vi "OP500Z8_SCANequipements.vi"(8 "Errin":errorcluster caption="errin", 10 "Chaîne":string="Log et conf\\Config.ini", 11 "pathin":path=path "D:/CODE/02 SLIM ZEN") -> (0 "errout":errorcluster={"status"=TRUE, "code"=0, "source"="PCAN_CHANNEL ILLEGAL"}, 1 "KO?":bool=TRUE, 3 "VISA OUT":T1)   [LabVIEW 2020]
doc: "Ce vi il détecte la presence des équipements"
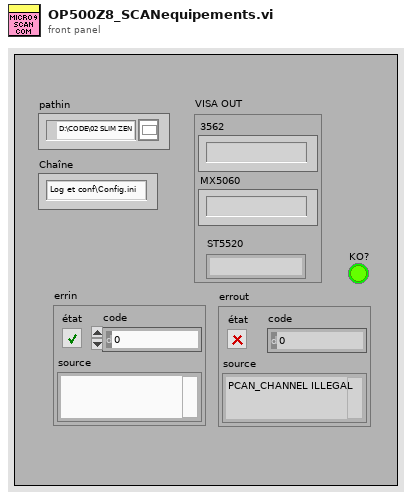
[diagram p1: front panel]
types:
  T1 = cluster{"3562":string, "MX5060":string, "ST5520":string}
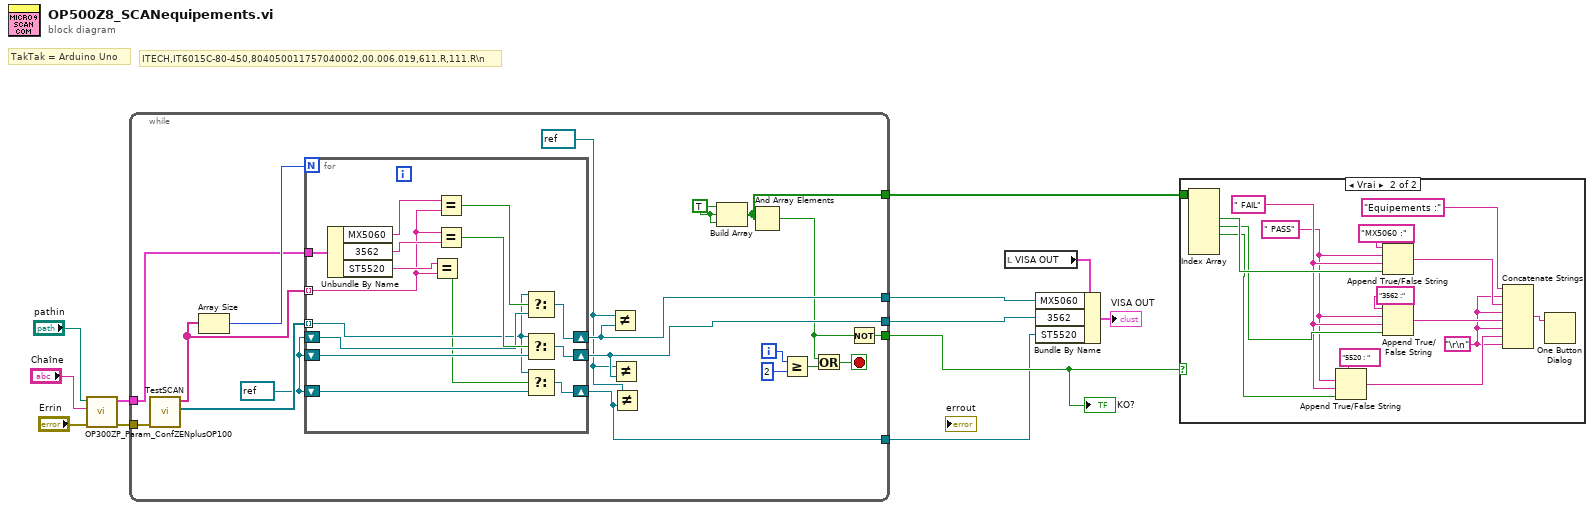
[diagram p0: block diagram]
diagram:
  # "TakTak = Arduino Uno"
  # "ITECH,IT6015C-80-450,804050011757040002,00.006.019,611.R,111.R\\n"
  n1 = call "OP300ZP_Param_ConfZENplusOP100.vi"("errin"="Errin", "Chaîne"="Chaîne", "pathin"="pathin") -> ("errout"=w7:errorcluster, "VISA OUT"=w6:T1)  [unwired: 7 in]
  n2 = while {
    tunnel: [w20] -> w12
    tunnel: [w19] -> w11
    tunnel: w7 -> [w29]
    tunnel: [w24] -> w10
    tunnel: w6 -> [w21]
    tunnel: [w17] -> w9
    tunnel: [w14] -> w1
    i -> [w23]
    stop <- w26 stop-if-true
    w13 = TRUE ("élément")
    w15 = refnum<visa-resource-name> refnum ("x")
    w16 = refnum<visa-resource-name> refnum ("VISA resource name out")
    n3 = call "TestSCAN.vi"("errin"=w29) -> ("Tableau 2"=w27:refnum<visa-resource-name>[], "Tableau"=w28:string[])  [unwired: 8 in, 1 out]
    n4 = Array Size(array=w28) -> (size(s)=w30:i32)
    n5 = for {
      N: w30 -> [_]
      shift-right: [w43] -> w20
      shift-left: w16 -> [w41]
      shift-right: [w42] -> w19
      shift-left: w16 -> [w40]
      tunnel: w28 -> [w32] mode=indexing
      tunnel: w21 -> [w39]
      shift-right: [w35] -> w14
      shift-left: w16 -> [w36]
      tunnel: w27 -> [w34] mode=indexing
      n6 = Unbundle By Name(w39) -> ("MX5060"=w38:string, "3562"=w37:string, "ST5520"=w33:string)
      n7 = Equal?(x=w33, y=w32) -> (x = y?=w31:bool)
      n8 = Equal?(x=w38, y=w32) -> (x = y?=w44:bool)
      n9 = Equal?(x=w32, y=w37) -> (x = y?=w45:bool)
      n10 = Select(t=w34, s=w44, f=w41) -> (s? t:f=w43:refnum<visa-resource-name>)
      n11 = Select(t=w34, s=w45, f=w40) -> (s? t:f=w42:refnum<visa-resource-name>)
      n12 = Select(t=w34, s=w31, f=w36) -> (s? t:f=w35:refnum<visa-resource-name>)
    }
    n13 = Not Equal?(x=w15, y=w20) -> ()  [unwired: 1 out]
    n14 = Not Equal?(x=w15, y=w19) -> ()  [unwired: 1 out]
    n15 = Not Equal?(x=w15, y=w14) -> ()  [unwired: 1 out]
    n16 = Build Array(w13, w13, w13) -> (w17:bool[])
    n17 = And Array Elements(Boolean array=w17) -> (logical AND=w18:bool)
    n18 = Greater Or Equal?(x=w23, y=2) -> (x >= y?=w25:bool)
    n19 = Or(x=w18, y=w25) -> (x .or. y?=w26:bool)
    n20 = Not(x=w18) -> (.not. x?=w24:bool)
  }
  "KO?" <- w10
  n21 = local read "VISA OUT"() -> (w2:T1)
  n22 = Bundle By Name(cluster=w2, "MX5060"=w12, "3562"=w11, "ST5520"=w1) -> (→"VISA OUT":T1)
  n23 = case shown="Vrai" w10 {
    tunnel: w9 -> [_ w51]
    frame False {
    }
    frame True {
      w52 = "\r\n"
      w46 = " PASS" ("chaîne faux")
      w47 = " FAIL" ("chaîne faux")
      n24 = Index Array(array=w51) -> (element #2=w50:bool, element #3=w49:bool, element #4=w48:bool)  [unwired: 6 in, 3 out]
      n25 = Append True/False String(1:w48, 2:w47, 3:w46, 4:"5520 : " ("chaîne (\"\")")) -> (0:w54:string)
      n26 = Append True/False String(1:w50, 2:w47, 3:w46, 4:"MX5060 :" ("chaîne (\"\")")) -> (0:w56:string)
      n27 = Append True/False String(1:w49, 2:w47, 3:w46, 4:"3562 :" ("chaîne (\"\")")) -> (0:w55:string)
      n28 = Concatenate Strings("Equipements :" ("chaîne"), w52, w56, w52, w55, w52, w54, w52) -> (w53:string)
      n29 = One Button Dialog(message=w53) -> ()  [unwired: 1 in, 1 out]
    }
  }
